vi "SQL_test_template_selete.vi"() -> (3 "表格控件":string[][](table))   [LabVIEW 2014]
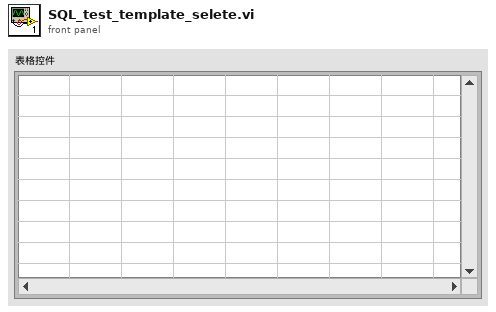
[diagram p1: front panel]
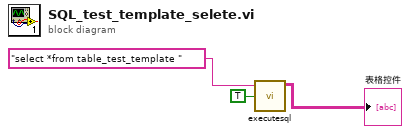
[diagram p0: block diagram]
diagram:
  n1 = call "executesql.vi"("Return Data (T)"=TRUE, "Command Text"="select *from table_test_template ") -> ("Data"=→"表格控件":string[][])  [unwired: 5 in, 1 out]
